vi "hysterisis.vi"(9 "cal_low":dbl, 10 "cal_high":dbl, 11 "input":dbl) -> (3 "output_latch":bool)   [LabVIEW 2013]
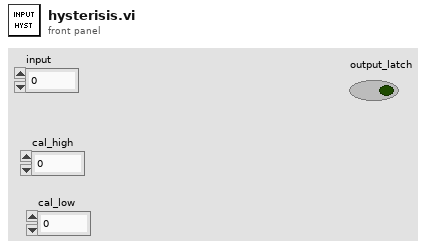
[diagram p1: front panel]
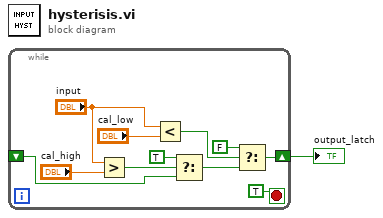
[diagram p0: block diagram]
diagram:
  n1 = while {
    shift-right: [w2] -> w1
    shift-left: _ -> [w7]
    stop <- TRUE stop-if-true
    n2 = Greater?(x="input", y="cal_high") -> (0:w8:bool)
    n3 = Less?(x="input", y="cal_low") -> (x < y?=w5:bool)
    n4 = Select(t=TRUE, s=w8, f=w7) -> (s? t:f=w4:bool)
    n5 = Select(t=FALSE, s=w5, f=w4) -> (s? t:f=w2:bool)
  }
  "output_latch" <- w1
